vi "while_v0_v11.vi"() -> ()   [LabVIEW 2009]
panel:
  in  "Delay":u8(slide)=52 scale=20.0..80.0
  in  "stop":bool
  out "Waveform Chart":dbl(graph)
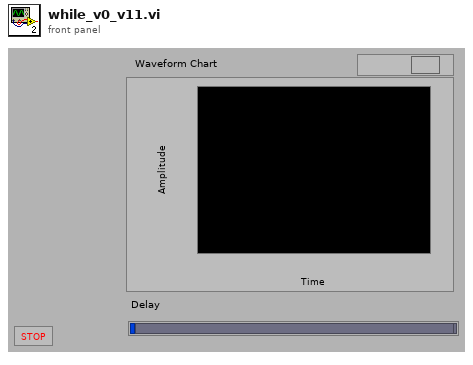
[diagram p1: front panel]
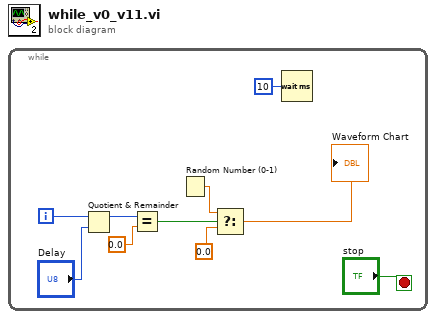
[diagram p0: block diagram]
diagram:
  n1 = while {
    i -> [w8]
    stop <- "stop" stop-if-true
    n2 = Quotient & Remainder(x=w8, y="Delay") -> (x-y*floor(x/y)=w4:i32)  [unwired: 1 out]
    n3 = Equal?(x=w4, y=0.0) -> (x = y?=w5:bool)
    n4 = Random Number (0-1)() -> (number: 0 to 1=w3:dbl)
    n5 = Select(t=w3, s=w5, f=0.0 ("t")) -> (s? t:f=→"Waveform Chart":dbl)
    n6 = Wait (ms)(milliseconds to wait=u32 10) -> ()  [unwired: 1 out]
  }
